vi "Find_File_Within_Folder.vi"(0 "Folder to Search":path, 1 "Files to find":path[](array[path])) -> (2 "Folder to Search Out":path, 3 "New File Paths":path[](array[path]), 4 "Files Found?":bool[](array[boolean]))   [LabVIEW 2010]
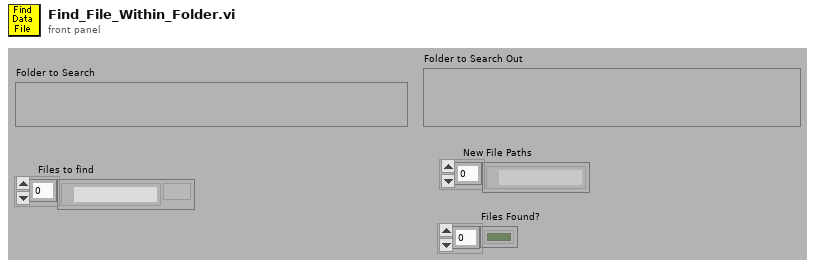
[diagram p1: front panel]
types:
  T1 = enum32{"existing file", "new file", "new or existing file", "existing dir", "new dir", "new or existing dir", "existing file (use LLBs)", "new file (use LLBs)", "new or existing file (use LLBs)", "new or existing file or directory (use LLBs)"}
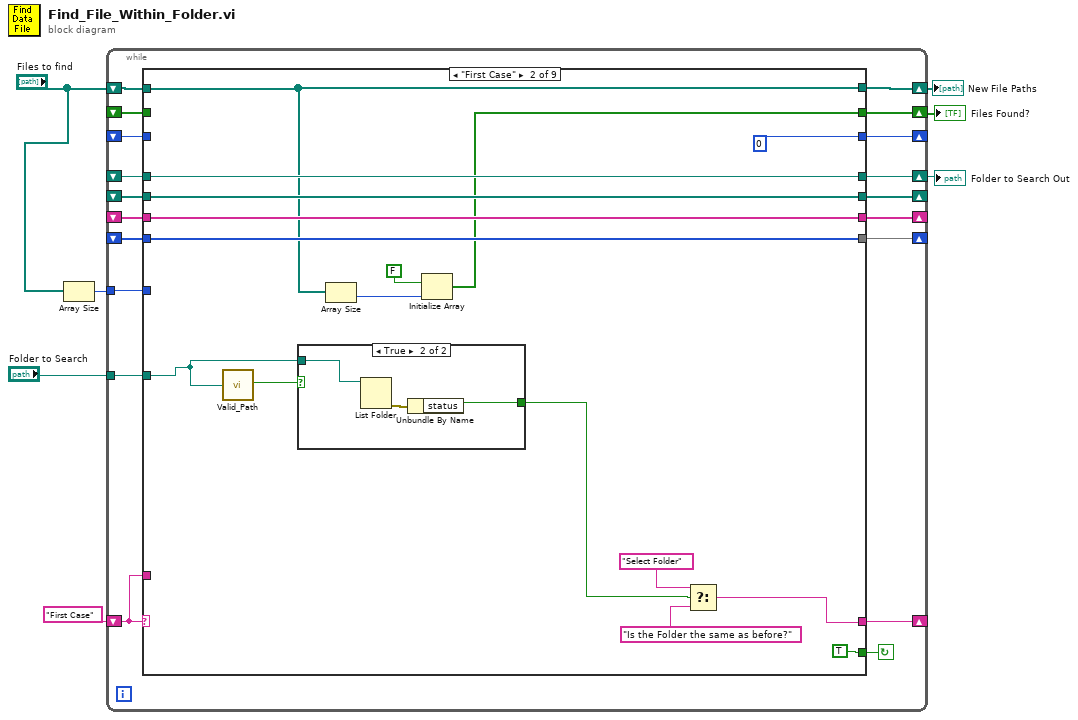
[diagram p0: block diagram]
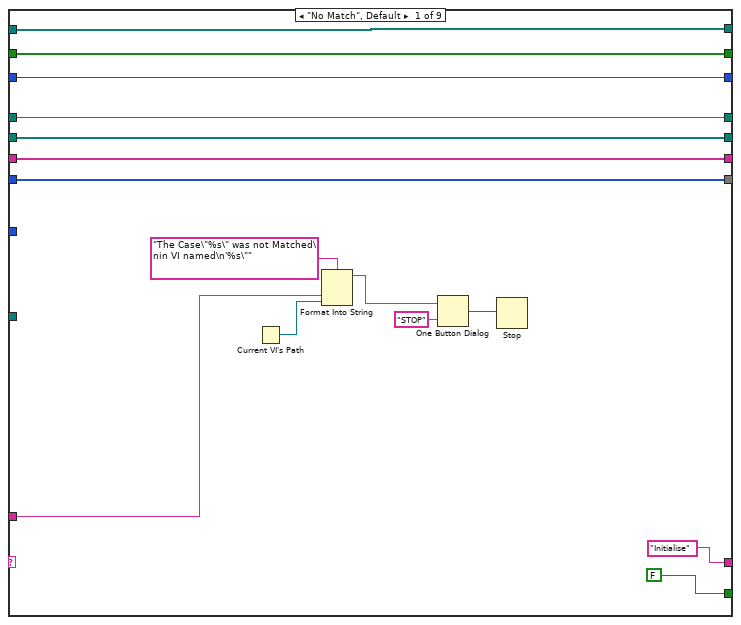
[diagram p2: hidden frame]
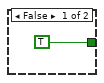
[diagram p3: hidden frame]
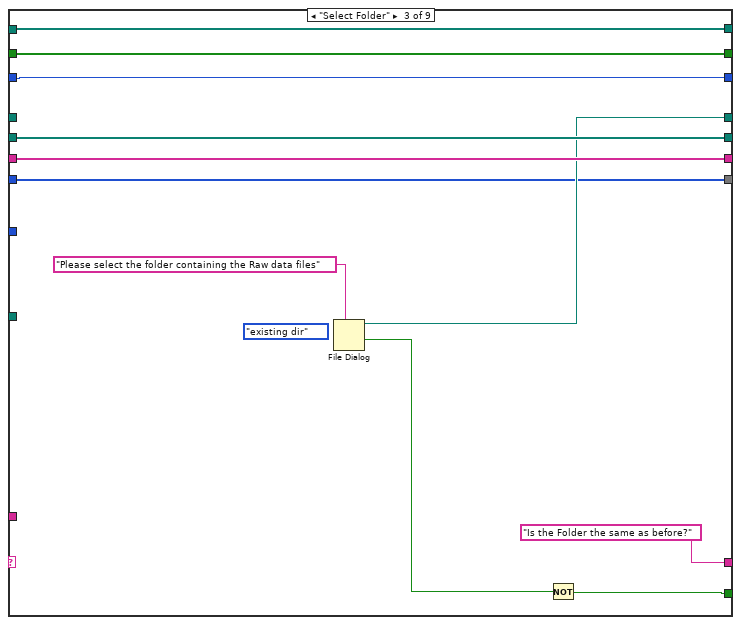
[diagram p4: hidden frame]
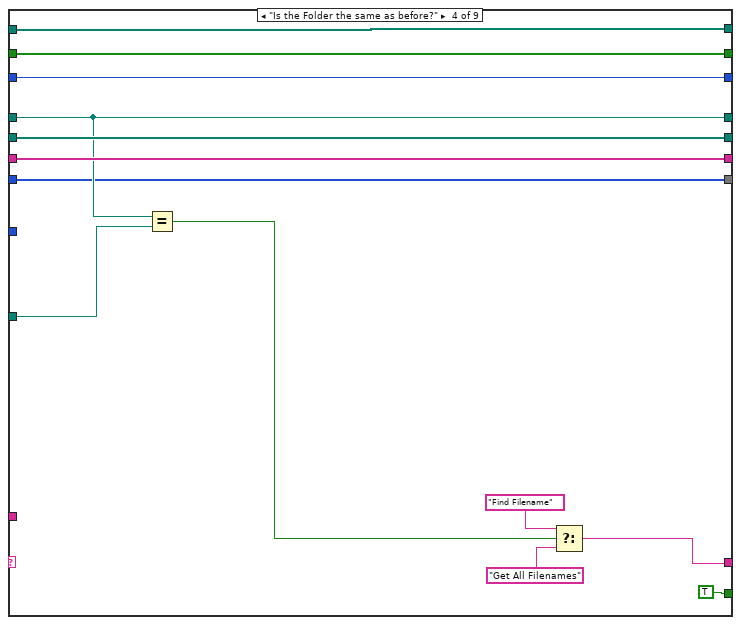
[diagram p5: hidden frame]
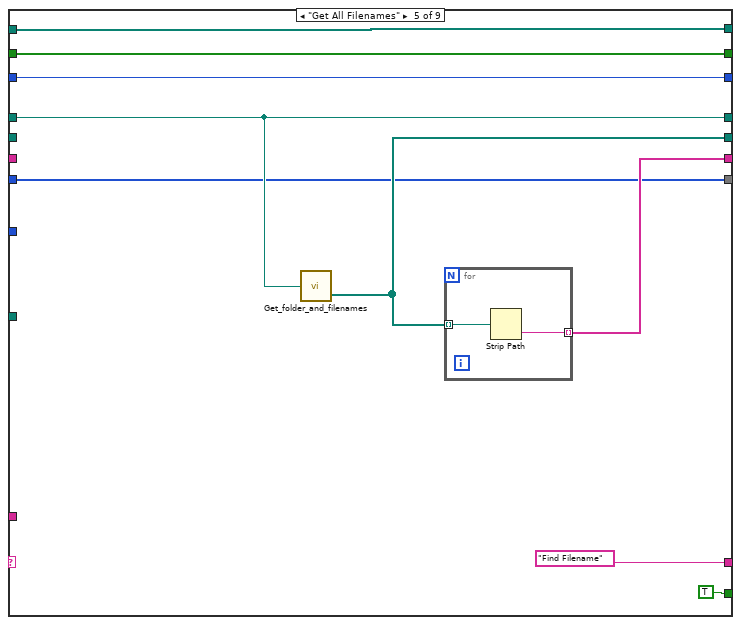
[diagram p6: hidden frame]
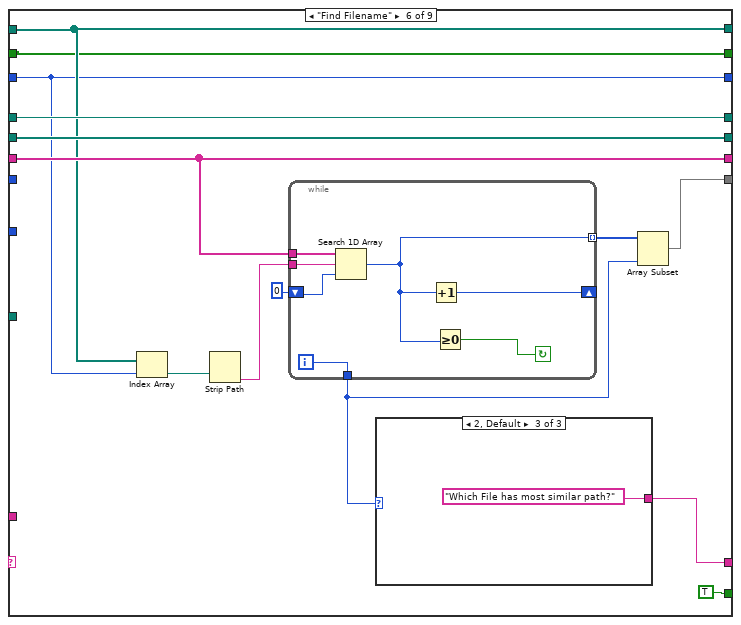
[diagram p7: hidden frame]
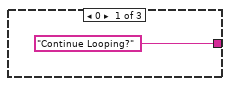
[diagram p8: hidden frame]
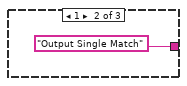
[diagram p9: hidden frame]
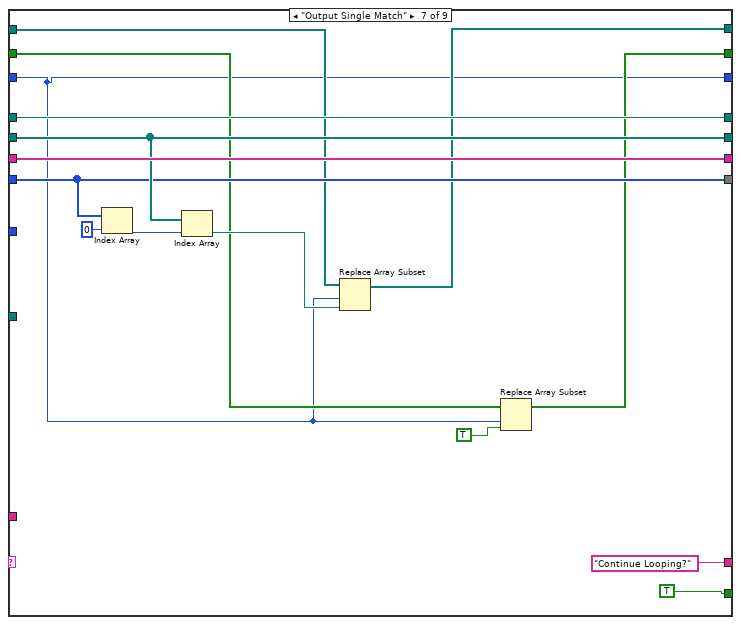
[diagram p10: hidden frame]
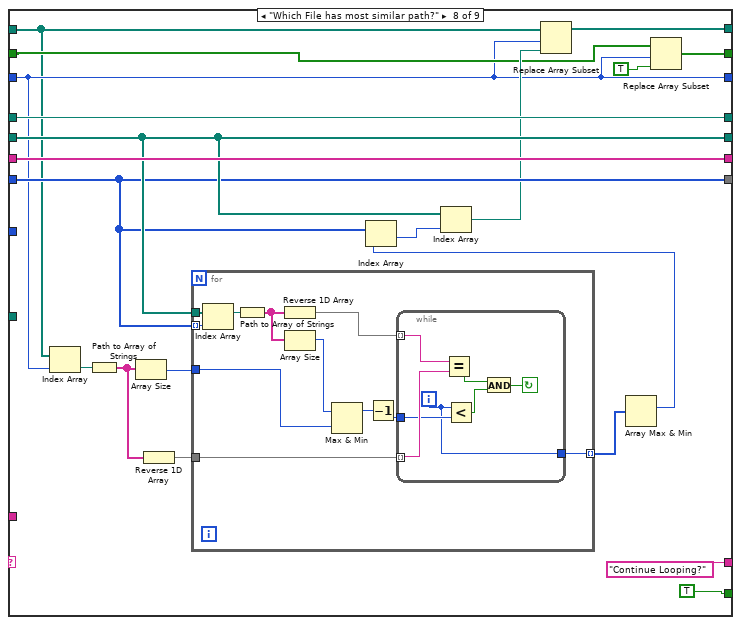
[diagram p11: hidden frame]
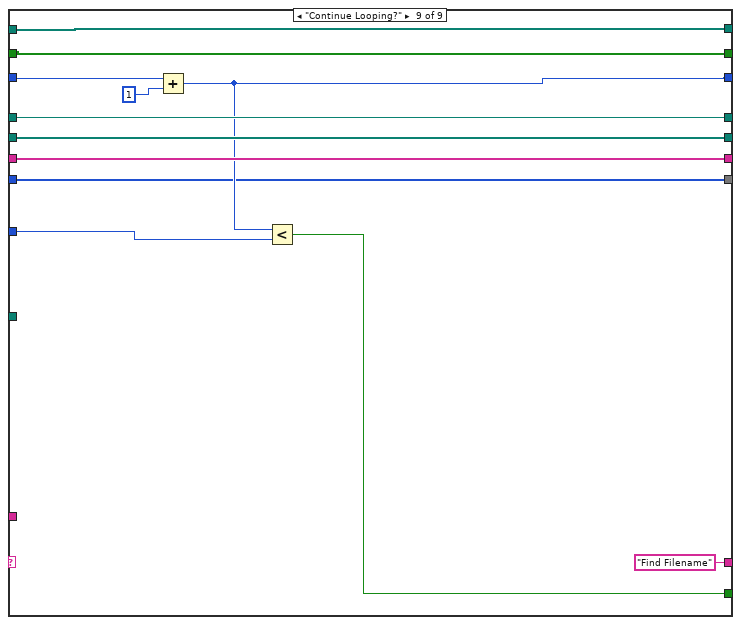
[diagram p12: hidden frame]
diagram:
  n1 = Array Size(array="Files to find") -> (size(s)=w1:i32)
  n2 = while {
    shift-left: _ -> [w15]
    shift-right: [w16] -> _
    tunnel: "Folder to Search" -> [w17]
    shift-left: _ -> [w19]
    shift-right: [w18] -> _
    shift-left: _ -> [w21]
    shift-right: [w20] -> _
    shift-left: _ -> [w23]
    shift-right: [w22] -> w5
    shift-left: "First Case" -> [w24]
    shift-right: [w25] -> _
    shift-right: [w14] -> _
    shift-left: _ -> [w9]
    shift-right: [w13] -> w3
    shift-left: _ -> [w10]
    shift-right: [w12] -> w4
    shift-left: "Files to find" -> [w11]
    tunnel: w1 -> [w8]
    stop <- w26 continue-if-true
    n3 = case shown="\"First Case\"" w24 {
      tunnel: [FALSE TRUE w72 TRUE TRUE TRUE TRUE TRUE w176] -> w26
      tunnel: ["Initialise" w54 "Is the Folder the same as before?" w82 "Find Filename" w101 "Continue Looping?" "Continue Looping?" "Find Filename"] -> w25
      tunnel: w24 -> [w36 _ _ _ _ _ _ _ _]
      tunnel: w23 -> [w33 w53 _ w77 w93 w105 w134 w154 w184]
      tunnel: [w33 w53 w68 w77 w93 w105 w134 w154 w184] -> w22
      tunnel: w21 -> [w32 w52 w71 w81 _ w109 w130 w150 w185]
      tunnel: [w32 w52 w71 w81 w92 w109 w130 w150 w185] -> w20
      tunnel: w19 -> [w31 w51 w70 w80 _ w108 w133 w153 w181]
      tunnel: [w31 w51 w70 w80 w91 w108 w133 w153 w181] -> w18
      tunnel: w17 -> [_ w43 _ w79 _ _ _ _ _]
      tunnel: [w30 w50 w67 w76 w89 w103 w128 w144 w174] -> w16
      tunnel: w15 -> [w30 w50 w67 w76 w89 _ w128 w144 w174]
      tunnel: [w27 0 w62 w73 w86 w97 w121 w138 w178] -> w14
      tunnel: [w28 w46 w63 w74 w87 w98 w123 w139 w183] -> w13
      tunnel: [w29 w45 w64 w75 w88 w99 w125 w143 w182] -> w12
      tunnel: w11 -> [w29 w45 w64 w75 w88 w99 w127 w137 w182]
      tunnel: w10 -> [w28 _ w63 w74 w87 w98 w124 w140 w183]
      tunnel: w9 -> [w27 _ w62 w73 w86 w97 w121 w138 w180]
      tunnel: w8 -> [_ _ _ _ _ _ _ _ w177]
      frame "No Match", Default {
        n4 = Current VI's Path() -> (path=w35:path)
        n5 = Format Into String(format string="The Case\"%s\" was not Matched\nin VI named\n'%s\"" ("Format String"), w36, w35) -> (resulting string=w39:string)  [unwired: 2 in, 1 out]
        n6 = One Button Dialog(message=w39, button name ("OK")="STOP") -> (true=w37:bool)
        n7 = Stop(stop? (T)=w37) -> ()
      }
      frame "First Case" {
        n8 = call "Valid_Path.vi"("Filename"=w43) -> ("Valid Path?"=w42:bool)
        n9 = case shown="True" w42 {
          tunnel: w43 -> [_ w61]
          tunnel: [TRUE w59] -> w44
          frame False {
          }
          frame True {
            n10 = List Folder(path=w61) -> (error out=w60:errorcluster)  [unwired: 1 in, 5 out]
            n11 = Unbundle By Name(w60) -> ("status"=w59:bool)
          }
        }
        n12 = Array Size(array=w45) -> (size(s)=w47:i32)
        n13 = Initialize Array(FALSE, w47) -> (w46:bool[])
        n14 = Select(t="Select Folder", s=w44, f="Is the Folder the same as before?") -> (s? t:f=w54:string)
      }
      frame "Select Folder" {
        (unwired) T1."existing dir" ("select mode (2)")
        n15 = File Dialog(7:"Please select the folder containing the Raw data files" ("prompt")) -> (1:w66:bool, 3:w68:path)  [unwired: 1 in, 7 out]
        n16 = Not(x=w66) -> (.not. x?=w72:bool)
      }
      frame "Is the Folder the same as before?" {
        n17 = Equal?(x=w77, y=w79) -> (x = y?=w78:bool)
        n18 = Select(t="Find Filename", s=w78, f="Get All Filenames") -> (s? t:f=w82:string)
      }
      frame "Get All Filenames" {
        n19 = call "Get_folder_and_filenames.vi"("file path (dialog if empty)"=w93) -> ("Files"=w92:path[])  [unwired: 1 out]
        n20 = for {
          tunnel: w92 -> [w96] mode=indexing
          tunnel: [w95] -> w91 mode=indexing
          n21 = Strip Path(path=w96) -> (name=w95:string)  [unwired: 1 out]
        }
      }
      frame "Find Filename" {
        n22 = Index Array(array=w99, index=w97) -> (element=w100:path)
        n23 = Strip Path(path=w100) -> (name=w107:string)  [unwired: 1 out]
        n24 = while {
          tunnel: [w111] -> w102
          tunnel: [w112] -> w104 mode=indexing
          shift-left: 0 -> [w115]
          shift-right: [w114] -> _
          tunnel: w107 -> [w116]
          tunnel: w108 -> [w117]
          i -> [w111]
          stop <- w113 continue-if-true
          n25 = Search 1D Array(1D array=w117, element=w116, start index (0)=w115) -> (index of element=w112:i32)
          n26 = Increment(x=w112) -> (x+1=w114:i32)
          n27 = Greater Or Equal To 0?(x=w112) -> (x >= 0?=w113:bool)
        }
        n28 = case shown="2, Default" w102 {
          tunnel: ["Continue Looping?" "Output Single Match" "Which File has most similar path?"] -> w101
          frame 0 {
          }
          frame 1 {
          }
          frame 2, Default {
          }
        }
        n29 = Array Subset(array=w104, length=w102) -> (w103:i32[])  [unwired: 1 in]
      }
      frame "Output Single Match" {
        n30 = Index Array(array=w128, index=0 ("Index")) -> (element=w131:i32)
        n31 = Index Array(array=w130, index=w131) -> (element=w126:path)
        n32 = Replace Array Subset(array=w127, new element=w126, index=w121) -> (w125:path[])
        n33 = Replace Array Subset(array=w124, new element=TRUE ("new element/subarray"), index=w121) -> (w123:bool[])
      }
      frame "Which File has most similar path?" {
        n34 = Index Array(array=w137, index=w138) -> (element=w136:path)
        n35 = Path to Array of Strings(0:w136) -> (2:w151:string[])  [unwired: 1 out]
        n36 = Array Size(array=w151) -> (size(s)=w149:i32)
        n37 = Reverse 1D Array(array=w151) -> (reversed array=w148:string[])
        n38 = for {
          tunnel: w150 -> [w161]
          tunnel: w144 -> [w160] mode=indexing
          tunnel: w149 -> [w158]
          tunnel: w148 -> [w157]
          tunnel: [w156] -> w147 mode=indexing
          n39 = Index Array(array=w161, index=w160) -> (element=w159:path)
          n40 = Path to Array of Strings(0:w159) -> (2:w165:string[])  [unwired: 1 out]
          n41 = Reverse 1D Array(array=w165) -> (reversed array=w164:string[])
          n42 = Array Size(array=w165) -> (size(s)=w166:i32)
          n43 = Max & Min(x=w166, y=w158) -> (max(x,y)=w163:i32)  [unwired: 1 out]
          n44 = Decrement(x=w163) -> (x-1=w162:i32)
          n45 = while {
            tunnel: [w167] -> w156
            tunnel: w162 -> [w171]
            tunnel: w157 -> [w172] mode=indexing
            tunnel: w164 -> [w173] mode=indexing
            i -> [w167]
            stop <- w169 continue-if-true
            n46 = Equal?(x=w173, y=w172) -> (x = y?=w168:bool)
            n47 = Less?(x=w167, y=w171) -> (x < y?=w170:bool)
            n48 = And(x=w168, y=w170) -> (x .and. y?=w169:bool)
          }
        }
        n49 = Array Max & Min(array=w147) -> (max index (indices)=w146:i32)  [unwired: 3 out]
        n50 = Index Array(array=w144, index=w146) -> (element=w145:i32)
        n51 = Index Array(array=w150, index=w145) -> (element=w142:path)
        n52 = Replace Array Subset(array=w137, new element=w142, index=w138) -> (w143:path[])
        n53 = Replace Array Subset(array=w140, new element=TRUE ("new element/subarray"), index=w138) -> (w139:bool[])
      }
      frame "Continue Looping?" {
        n54 = Add(x=w180, y=1) -> (x+y=w178:i32)
        n55 = Less?(x=w178, y=w177) -> (x < y?=w176:bool)
      }
    }
  }
  "Folder to Search Out" <- w5
  "New File Paths" <- w4
  "Files Found?" <- w3
